vi "serial_AUCT.vi"() -> ()   [LabVIEW 2018]
uses:
  Controls created/Control 3.ctl
  Controls created/Control 4.ctl
  <vilib>/Instr/_visa.llb/VISA Configure Serial Port (Instr).vi
  <instrlib>/LeCroy Wave Series/Public/Data/Read Single Waveform.vi
  <instrlib>/Siglent SDG X Series/Siglent SDG X Series.lvlib
  <instrlib>/LeCroy Wave Series/LeCroy Wave Series.lvlib
panel:
  in  "Tab Control":enum32{"Page 1", "Page 2", "Page 3"}(tab)
  in  "VISA resource":refnum<visa-resource-name>
  in  "NR":i16=1600
  in  "Set Speed (Steps/s)":i16=1200 min=0 max=3000 step=50
  in  "Baud Rate":u32=115200
  out "Iteration #":i32
  in  "NT":i16
  out "Error":errorcluster
  in  "Arbitray Movement":bool
  out "stop motion":bool
  in  "MOTION":bool
  in  "?":i8(slide) step=2 scale=0.0..2.0
  in  "OK Button":bool
  out "# NT":i32
  in  "Scanning Distance\n(in mm)":i32
  in  "ms to wait(Translation)":u32
  out "Dis_step":dbl
  in  "milliseconds to wait":u32
  in  "ms to wait(Rotation)":u32
  in  "VISA Refnum in":refnum<visa-resource-name>="USB0::0xF4EC::0xEE38::SDG2XCAD2R3765::INSTR"
  in  "Channel (1:Channel 1)":i32(ring)=1 items=["Channel 1"=1, "Channel 2"=2]
  in  "Enable Output (T: Enable)":bool=TRUE
  in  "Amplitude (1.0 Vpp)":dbl=20.0 format="%#.3f"
  in  "Frequency (1000 Hz)":T1=1500000.0 format="%#.6g"
  in  "DC Offset (0.00 V) in":dbl
  in  "Waveform Function (0: Sine) in":u16(ring) items=["Sine", "Square", "Ramp", "DC", "Pulse", "Arb"]
  in  "Phase (0.0 degrees)":dbl=0.002 min=-360.0 max=360.0 format="%#.1g"
  in  "Fall (20 ns)":dbl=8.4e-09 format="%#.3g"
  in  "Duty (20%)":dbl=4.32 min=0.0001 max=100.0 format="%.4g"
  in  "Delay (0.00 s)":dbl min=-1000000.0 max=1000000.0
  in  "Rise (20 ns)":dbl=1.04e-08 format="%#.3g"
  in  "True To \ngenerate\n pulse":T2=TRUE
  out "VISA resource name out":refnum<visa-resource-name>
  out "error out":errorcluster
  out "Output Filename":path
  out "error out 2":errorcluster
  in  "format string":string="Channel: %g \nWavetype: %g \nAMP: %gV\nFreq: %gHz \nRiseTime: %gs \nFallTime: %gs \nDutyCycle: %g"
  out "Output Directory":path
  in  "File Directory":path=path "E:/Ankur/Labview/Automation/Data/Exp1"
  in  "Filename 2":string
  out "Oscilloscope\n Runnning":bool
  in  "stop":bool
  out "Waveform Data":waveform(dbl)(graph)
  in  "Timeout (10000 ms)":u32=10000
  in  "Source (0: Channel 1)":u16(ring) items=["Channel 1", "Channel 2", "Channel 3", "Channel 4", "Memory 1", "Memory 2", "Memory 3", "Memory 4", "Function 1", "Function 2", "Function 3", "Function 4", "Function 5", "Function 6", "Function 7", "Function 8"]
  in  "Perform Auto Setup?":bool
  in  "Reset Scope?":bool
  in  "VISA resource name":refnum<visa-resource-name>="LecroyHDO4024-1"
  in  "Save Files in Directory (In Oscilloscope)":string="D:\\Automation\\Data"
  in  "Filename":string="Title"
  in  "Path to save DATA":path=path "E:/Ankur/Labview/Automation/Files/Oscdata"
  out "Saved filename":string
  in  "Save File locally":bool
  # "For Rotational motion"
  # "For Translational Motion"
  # "For Translational motion"
  # "OFF"
  # "ON"
  # "Yes"
  # "No"
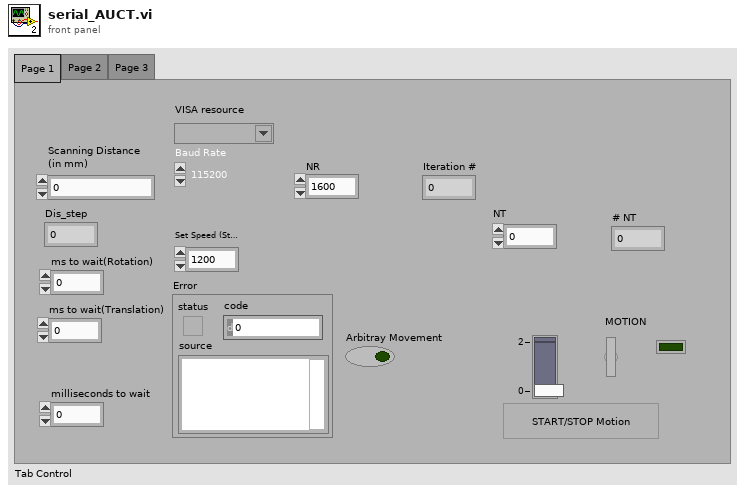
[diagram p1: front panel]
types:
  T1 = typedef "Control 3.ctl" = dbl
  T2 = typedef "Control 4.ctl" = bool
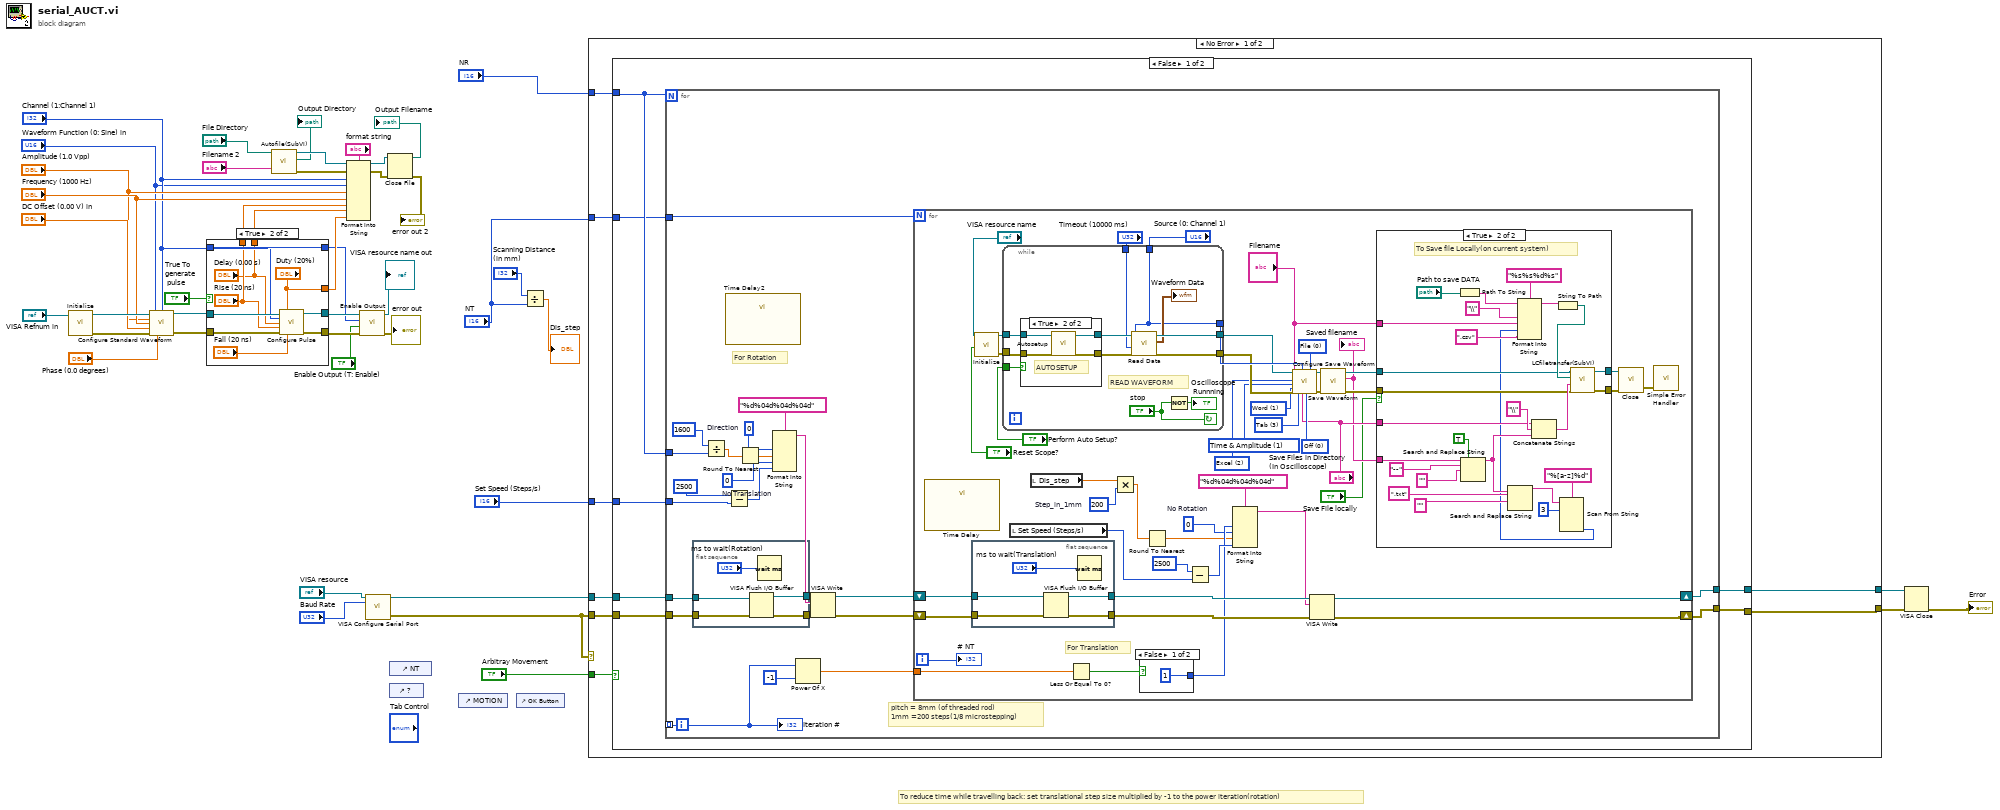
[diagram p0: block diagram]
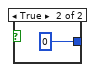
[diagram p2: hidden frame]
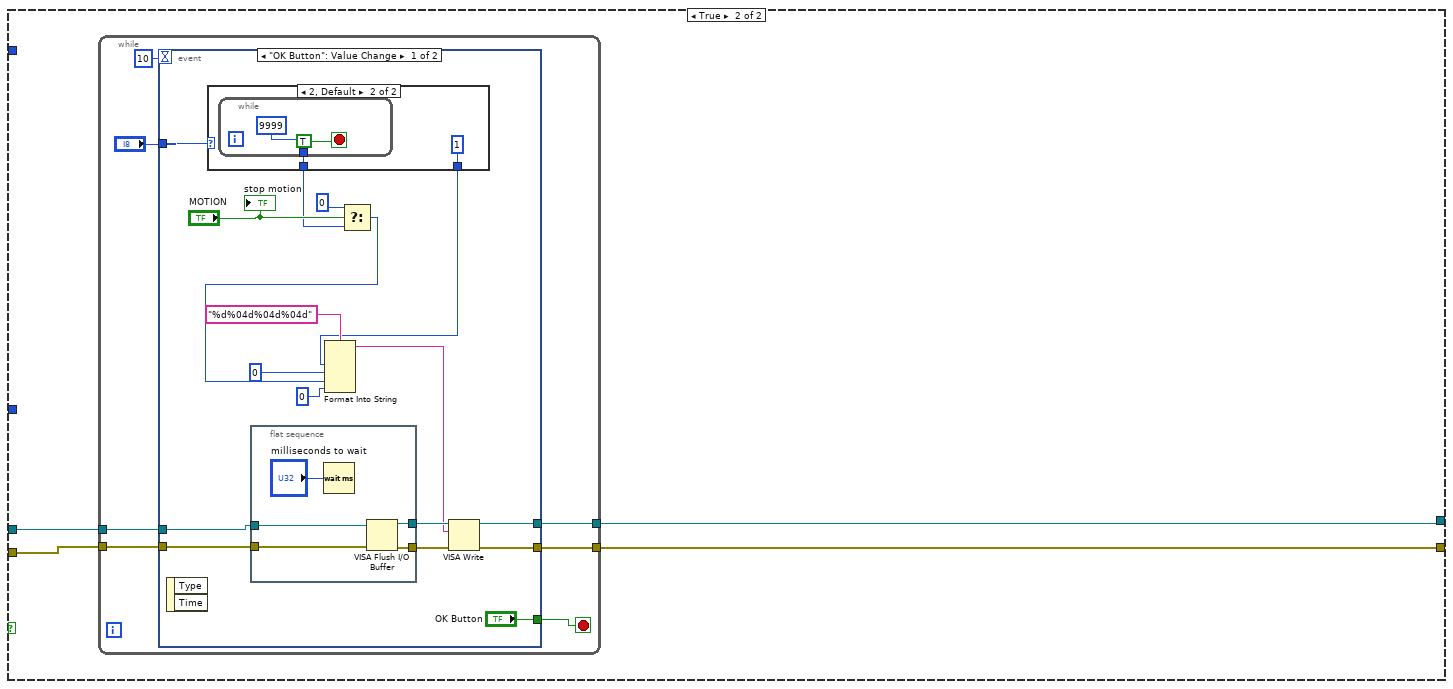
[diagram p5: hidden frame]
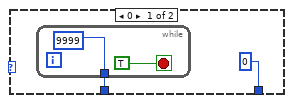
[diagram p6: hidden frame]
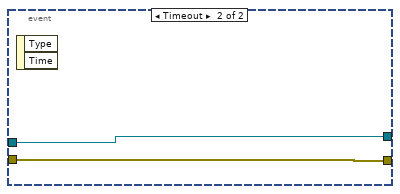
[diagram p7: hidden frame]
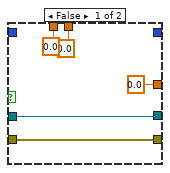
[diagram p9: hidden frame]
diagram:
  # "To reduce time while travelling back: set translational step size multiplied by -1 to the power iteration(rotation)"
  n1 = call <instrlib>:"Initialize.vi"("VISA resource name"="VISA Refnum in") -> ("error out"=w35:errorcluster, "VISA resource name out"=w36:refnum<visa-resource-name>)  [unwired: 9 in]
  n2 = call <instrlib>:"Configure Standard Waveform.vi"("VISA resource name"=w36, "Waveform Function (0: Sine)"="Waveform Function (0: Sine) in", "Channel (1:Channel 1)"="Channel (1:Channel 1)", "Amplitude (1.0 Vpp)"="Amplitude (1.0 Vpp)", "Frequency (1000 Hz)"="Frequency (1000 Hz)", "DC Offset (0.00 V)"="DC Offset (0.00 V) in", "error in (no error)"=w35, "Phase (0.0 degrees)"="Phase (0.0 degrees)") -> ("VISA resource name out"=w31:refnum<visa-resource-name>, "error out"=w34:errorcluster)  [unwired: 6 in]
  n3 = case shown="True" "True To \ngenerate\n pulse" {
    tunnel: [w48 w56] -> w40
    tunnel: [w47 w55] -> w39
    tunnel: w31 -> [w48 w54]
    tunnel: w34 -> [w47 w53]
    tunnel: "Channel (1:Channel 1)" -> [_ w52]
    tunnel: "Channel (1:Channel 1)" -> [_ _]
    tunnel: [0.0 ("Duty (20%)") "Duty (20%)"] -> w27
    tunnel: [0.0 ("Rise (20 ns)") "Rise (20 ns)"] -> w19
    tunnel: [0.0 ("Delay (0.00 s)") "Delay (0.00 s)"] -> w18
    frame False {
    }
    frame True {
      n4 = call <instrlib>:"Configure Pulse.vi"("VISA resource name"=w54, "Duty (20%)"="Duty (20%)", "Channel (1:Channel 1)"=w52, "Delay (0.00 s)"="Delay (0.00 s)", "Rise (20 ns)"="Rise (20 ns)", "error in (no error)"=w53, "Fall (20 ns)"="Fall (20 ns)") -> ("VISA resource name out"=w56:refnum<visa-resource-name>, "error out"=w55:errorcluster)  [unwired: 7 in]
    }
  }
  n5 = call "Autofile(SubVI).vi"("Filename"="Filename 2", "File Directory"="File Directory") -> ("error out"=w14:errorcluster, "Output Directory"=→"Output Directory":path, "Byte Stream File out"=w15:refnum<file>)  [unwired: 7 in]
  n6 = Format Into String(format string="format string", initial string=w15, error in=w14, "Channel (1:Channel 1)", "Waveform Function (0: Sine) in", "Amplitude (1.0 Vpp)", "Frequency (1000 Hz)", w19, w18, w27) -> (resulting string=w26:refnum<file>, error out=w23:errorcluster)
  n7 = call <instrlib>:"Enable Output.vi"("error in (no error)"=w39, "Enable Output (T: Enable)"="Enable Output (T: Enable)", "Channel (1:Channel 1)"="Channel (1:Channel 1)", "VISA resource name"=w40) -> ("error out"=→"error out":errorcluster, "VISA resource name out"=→"VISA resource name out":refnum<visa-resource-name>)  [unwired: 6 in]
  n8 = call-poly "VISA Configure Serial Port"("VISA resource name"="VISA resource", "baud rate (9600)"="Baud Rate") -> ("VISA resource name out"=w7:refnum<visa-resource-name>, "error out"=w8:errorcluster)  [unwired: 12 in]
  n9 = Close File(refnum=w26, error in=w23) -> (path=→"Output Filename":path, error out=→"error out 2":errorcluster)
  n10 = control-ref of="NT"() -> ()  [unwired: 1 out]
  n11 = control-ref of="?"() -> ()  [unwired: 1 out]
  n12 = control-ref of="MOTION"() -> ()  [unwired: 1 out]
  n13 = control-ref of="OK Button"() -> ()  [unwired: 1 out]
  n14 = Divide(x="Scanning Distance\n(in mm)", y="NT") -> (x/y=→"Dis_step":dbl)
  n15 = case shown="No Error" w8 {
    tunnel: [w58 w245] -> w4
    tunnel: "NR" -> [w65 _]
    tunnel: "Set Speed (Steps/s)" -> [w64 _]
    tunnel: "Arbitray Movement" -> [w63 _]
    tunnel: w8 -> [w62 w245]
    tunnel: w7 -> [w61 w244]
    tunnel: "NT" -> [w60 _]
    tunnel: [w59 w244] -> w1
    frame No Error {
      n16 = case shown="False" w63 {
        tunnel: w65 -> [w69 _]
        tunnel: w64 -> [w72 _]
        tunnel: w62 -> [w71 w204]
        tunnel: w61 -> [w70 w203]
        tunnel: w60 -> [w68 _]
        tunnel: [w67 w202] -> w59
        tunnel: [w66 w201] -> w58
        frame False {
          n17 = for {
            N: w69 -> [_]
            tunnel: [w92] -> w66
            tunnel: [w93] -> w67
            tunnel: w72 -> [w73]
            tunnel: [w95] -> _ mode=indexing
            tunnel: w71 -> [w86]
            tunnel: w70 -> [w87]
            tunnel: w69 -> [w79]
            tunnel: w68 -> [w75]
            i -> [w95]
            w83 = 0  # No Translation
            w81 = 0  # Direction
            # "pitch = 8mm (of threaded rod)\n1mm =200 steps(1/8 microstepping)"
            # "For Rotation"
            n18 = flat-sequence {
              tunnel: [w100] -> w90
              tunnel: [w99] -> w91
              tunnel: w87 -> [w97]
              tunnel: w86 -> [w96]
              frame #0 {
                n19 = VISA Flush I/O Buffer(VISA resource name=w97, error in (no error)=w96) -> (VISA resource name out=w100:refnum<visa-resource-name>, error out=w99:errorcluster)  [unwired: 1 in]
                n20 = Wait (ms)(milliseconds to wait="ms to wait(Rotation)") -> ()  [unwired: 1 out]
              }
            }
            n21 = Divide(x=i16 1600, y=w79) -> (x/y=w78:dbl)
            n22 = call "Time Delay2"() -> ()  [unwired: 11 in, 1 out]
            n23 = Subtract(x=i16 2500 ("y"), y=w73) -> (x-y=w82:i16)
            n24 = Round To Nearest(number=w78) -> (nearest integer value=w77:dbl)
            n25 = Format Into String(format string="%d%04d%04d%04d", w81, w77, w83, w82) -> (resulting string=w85:string)  [unwired: 2 in, 1 out]
            n26 = Power Of X(1:-1 ("x"), 2:w95) -> (0:w76:dbl)
            n27 = VISA Write(VISA resource name=w90, write buffer=w85, error in (no error)=w91) -> (VISA resource name out=w88:refnum<visa-resource-name>, error out=w89:errorcluster)  [unwired: 1 out]
            n28 = for {
              N: w75 -> [_]
              shift-right: [w109] -> w93
              shift-left: w88 -> [w119]
              shift-right: [w108] -> w92
              shift-left: w89 -> [w118]
              tunnel: w76 -> [w112]
              i -> [w147]
              w104 = 200  # Step_in_1mm
              w107 = 0  # No Rotation
              w133 = u16 3 items=["Comma", "Space", "Semicolon", "Tab"] ("Delimiter (  0:Comma)")
              w132 = u16 0 items=["Off", "Wrap", "Fill"] ("Auto Save (0:Off")
              w134 = u16 1 items=["Byte", "Word", "Auto"] ("BinarySubFormat (1: Word)")
              w135 = u16 1 items=["Amplitude Only", "Time & Amplitude", "With Header"] ("SubFormat (1: Time & Amplitude)")
              w136 = u16 2 items=["Binary", "ASCII", "Excel", "MATLAB", "MathCad", "WaveML"] ("Format (0: Binary)")
              w131 = u16 0 items=["File", "M1", "M2", "M3", "M4"] ("Destination (0:File)")
              # "For Translation"
              n29 = call "Time Delay"() -> ()  [unwired: 11 in, 1 out]
              n30 = flat-sequence {
                tunnel: [w154] -> w117
                tunnel: [w153] -> w116
                tunnel: w119 -> [w151]
                tunnel: w118 -> [w150]
                frame #0 {
                  n31 = VISA Flush I/O Buffer(VISA resource name=w151, error in (no error)=w150) -> (VISA resource name out=w154:refnum<visa-resource-name>, error out=w153:errorcluster)  [unwired: 1 in]
                  n32 = Wait (ms)(milliseconds to wait="ms to wait(Translation)") -> ()  [unwired: 1 out]
                }
              }
              n33 = call <instrlib>:"Initialize.vi"("Reset? (T: Yes)"="Reset Scope?", "VISA resource name"="VISA resource name") -> ("error out"=w139:errorcluster, "VISA resource name out"=w138:refnum<visa-resource-name>)  [unwired: 8 in]
              n34 = while {
                tunnel: [w192] -> w145
                tunnel: [w191] -> w144
                tunnel: "Perform Auto Setup?" -> [w190]
                tunnel: "Source (0: Channel 1)" -> [w183]
                tunnel: w139 -> [w189]
                tunnel: w138 -> [w188]
                tunnel: "Timeout (10000 ms)" -> [w187]
                tunnel: [w183] -> w146
                stop <- "stop" continue-if-true
                # "READ WAVEFORM"
                n35 = case shown="True" w190 {
                  tunnel: w189 -> [w195 w200]
                  tunnel: w188 -> [w196 w199]
                  tunnel: [w196 w198] -> w194
                  tunnel: [w195 w197] -> w193
                  frame False {
                  }
                  frame True {
                    # "AUTOSETUP"
                    n36 = call <instrlib>:"Autosetup.vi"("error in (no error)"=w200, "VISA resource name"=w199) -> ("error out"=w197:errorcluster, "VISA resource name out"=w198:refnum<visa-resource-name>)  [unwired: 8 in]
                  }
                }
                n37 = call-poly <instrlib>:"Read Data.vi"("error in (no error)"=w193, "Timeout (10000 ms)"=w187, "Source (0: Channel 1)"=w183, "VISA resource name"=w194) -> ("error out"=w192:errorcluster, "Waveform Data"=→"Waveform Data":waveform(dbl), "VISA resource name out"=w191:refnum<visa-resource-name>)  [unwired: 5 in]
                n38 = Not(x="stop") -> (.not. x?=→"Oscilloscope\n Runnning":bool)
              }
              n39 = local read "Set Speed (Steps/s)"() -> (w101:i16)
              n40 = local read "Dis_step"() -> (w105:dbl)
              n41 = Less Or Equal To 0?(x=w112) -> (x <= 0?=w111:bool)
              n42 = Multiply(x=w105, y=w104) -> (x*y=w103:dbl)
              n43 = case shown="False" w111 {
                tunnel: [1 0] -> w110
                frame False {
                }
                frame True {
                }
              }
              n44 = Round To Nearest(number=w103) -> (nearest integer value=w106:dbl)
              n45 = Subtract(x=i16 2500 ("y"), y=w101) -> (x-y=w115:i16)
              n46 = Format Into String(format string="%d%04d%04d%04d", w110, w107, w106, w115) -> (resulting string=w113:string)  [unwired: 2 in, 1 out]
              n47 = call <instrlib>:"Configure Save Waveform.vi"("VISA resource name"=w144, "Trace Title (Title)"="Filename", "Format (0: Binary)"=w136, "SubFormat (1: Time & Amplitude)"=w135, "BinarySubFormat (1: Word)"=w134, "error in (no error)"=w145, "Delimiter (  0:Comma)"=w133, "Source (0: Channel 1)"=w146, "Save Files in Directory (D:\\Waveforms)"="Save Files in Directory (In Oscilloscope)", "Auto Save (0:Off"=w132, "Destination (0:File)"=w131) -> ("VISA resource name out"=w130:refnum<visa-resource-name>, "error out"=w129:errorcluster)  [unwired: 7 in]
              n48 = VISA Write(VISA resource name=w117, write buffer=w113, error in (no error)=w116) -> (VISA resource name out=w109:refnum<visa-resource-name>, error out=w108:errorcluster)  [unwired: 1 out]
              n49 = call <instrlib>:"Save Waveform.vi"("error in (no error)"=w129, "VISA resource name"=w130) -> ("error out"=w124:errorcluster, "Saved filename"=w122:string, "VISA resource name out"=w123:refnum<visa-resource-name>)  [unwired: 7 in]
              "Saved filename" <- w122
              n50 = case shown="True" "Save File locally" {
                tunnel: [w156 w179] -> w127
                tunnel: [w155 w178] -> w126
                tunnel: "Save Files in Directory (In Oscilloscope)" -> [_ w172]
                tunnel: w124 -> [w155 w171]
                tunnel: w123 -> [w156 w170]
                tunnel: w122 -> [_ w169]
                tunnel: "Filename" -> [_ w168]
                frame False {
                }
                frame True {
                  # "To Save file Locally(on current system)"
                  n51 = Path To String(path="Path to save DATA") -> (string=w173:string)
                  n52 = Search and Replace String(replace all?=TRUE ("replace all? (F)"), input string=w169, search string="--", replace string="" ("replace string (\"\")")) -> (result string=w164:string)  [unwired: 4 in, 3 out]
                  n53 = Search and Replace String(input string=w164, search string=".txt", replace string="" ("replace string (\"\")")) -> (result string=w167:string)  [unwired: 5 in, 3 out]
                  n54 = Concatenate Strings(w172, "\\" ("string"), w164) -> (w180:string)
                  n55 = Scan From String(format string="%[a-z]%d", input string=w167, initial scan location=u32 3) -> (output 2=w160:i32)  [unwired: 4 in, 3 out]
                  n56 = Format Into String(format string="%s%s%d%s", initial string=w173, "\\" ("input 1"), w168, w160, ".csv" ("input 3")) -> (resulting string=w159:string)  [unwired: 1 in, 1 out]
                  n57 = String To Path(string=w159) -> (path=w177:path)
                  n58 = call <userlib>:"LCfiletransfer(SubVI).vi"("error in (no error)"=w171, "Source Filename"=w180, "file path (use dialog)"=w177, "VISA Refnum in"=w170) -> ("error out"=w178:errorcluster, "VISA Refnum out"=w179:refnum<visa-resource-name>)  [unwired: 5 in, 1 out]
                }
              }
              n59 = call <instrlib>:"Close.vi"("error in (no error)"=w126, "VISA resource name"=w127) -> ("error out"=w128:errorcluster)  [unwired: 9 in]
              n60 = call <vilib>:"Simple Error Handler.vi"("error in (no error)"=w128) -> ()  [unwired: 4 in, 5 out]
              "# NT" <- w147
            }
            "Iteration #" <- w95
          }
        }
        frame True {
          n61 = while {
            tunnel: w204 -> [w209]
            tunnel: w203 -> [w208]
            tunnel: [w206] -> w202
            tunnel: [w207] -> w201
            stop <- w205 stop-if-true
            n62 = event shown="[0] \"OK Button\": Value Change" {
              selector: _ -> [_ _]
              dyn-events: _ -> [_ _]
              timeout: 10 -> [_ _]
              tunnel: "?" -> [w227 _]
              tunnel: w209 -> [w217 w242]
              tunnel: w208 -> [w218 w243]
              tunnel: [w215 w242] -> w207
              tunnel: [w216 w243] -> w206
              tunnel: ["OK Button" _] -> w205
              event "OK Button": Value Change {
                n63 = event-data() -> ()  [unwired: 1 in, 2 out]
                n64 = case shown="2, Default" w227 {
                  tunnel: [w235 w239] -> w225
                  tunnel: [0 ("input 1") 1 ("input 1")] -> w213
                  frame 0 {
                    n65 = while {
                      tunnel: [i16 9999 ("# of Steps to Move")] -> w235
                      stop <- TRUE ("Stop Reverse movement") stop-if-true
                    }
                  }
                  frame 2, Default {
                    n66 = while {
                      tunnel: [i16 9999 ("# of Steps to Move")] -> w239
                      stop <- TRUE ("Stop Forward movement") stop-if-true
                    }
                  }
                }
                n67 = flat-sequence {
                  tunnel: [w233] -> w224
                  tunnel: [w232] -> w223
                  tunnel: w218 -> [w230]
                  tunnel: w217 -> [w229]
                  frame #0 {
                    n68 = Wait (ms)(milliseconds to wait="milliseconds to wait") -> ()  [unwired: 1 out]
                    n69 = VISA Flush I/O Buffer(VISA resource name=w230, error in (no error)=w229) -> (VISA resource name out=w233:refnum<visa-resource-name>, error out=w232:errorcluster)  [unwired: 1 in]
                  }
                }
                n70 = Select(t=0, s="MOTION", f=w225) -> (s? t:f=w214:i32)
                n71 = Format Into String(format string="%d%04d%04d%04d", w213, 0 ("input 2"), w214, 0 ("input 4")) -> (resulting string=w221:string)  [unwired: 2 in, 1 out]
                n72 = VISA Write(VISA resource name=w224, write buffer=w221, error in (no error)=w223) -> (VISA resource name out=w216:refnum<visa-resource-name>, error out=w215:errorcluster)  [unwired: 1 out]
                "stop motion" <- "MOTION"
              }
              event Timeout {
                n73 = event-data() -> ()  [unwired: 1 in, 2 out]
              }
            }
          }
        }
      }
    }
    frame Error {
    }
  }
  n74 = VISA Close(VISA resource name=w1, error in (no error)=w4) -> (error out=→"Error":errorcluster)
